vi "WS1050 Delta C Calculation.vi"(7 "WS1050/51":bool=TRUE, 8 "error in (no error)":errorcluster, 10 "DCap Target(pF)":dbl, 11 "Input":string[][](table)) -> (0 "error out":errorcluster, 1 "Total Bank Delta C(pF)":string[](array[string]), 2 "RTZ(pF)":string[][](array[string]), 3 "Delta C(pF)":string[][](array[string]), 4 "% Bank DeltaC":string[](array[string]))   [LabVIEW 2012]
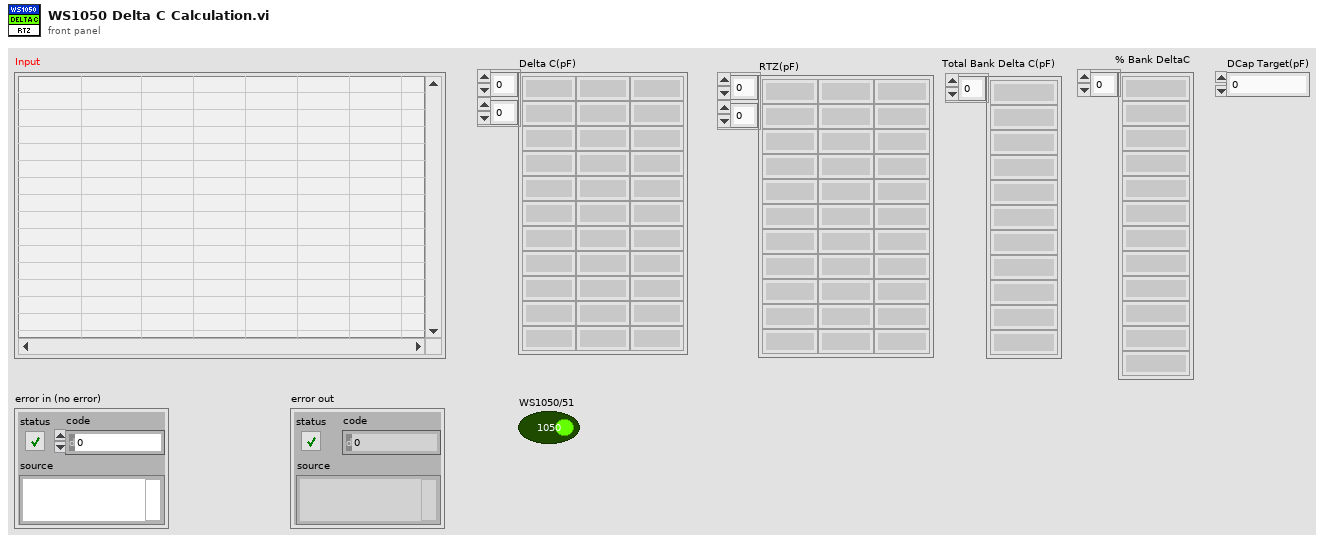
[diagram p1: front panel]
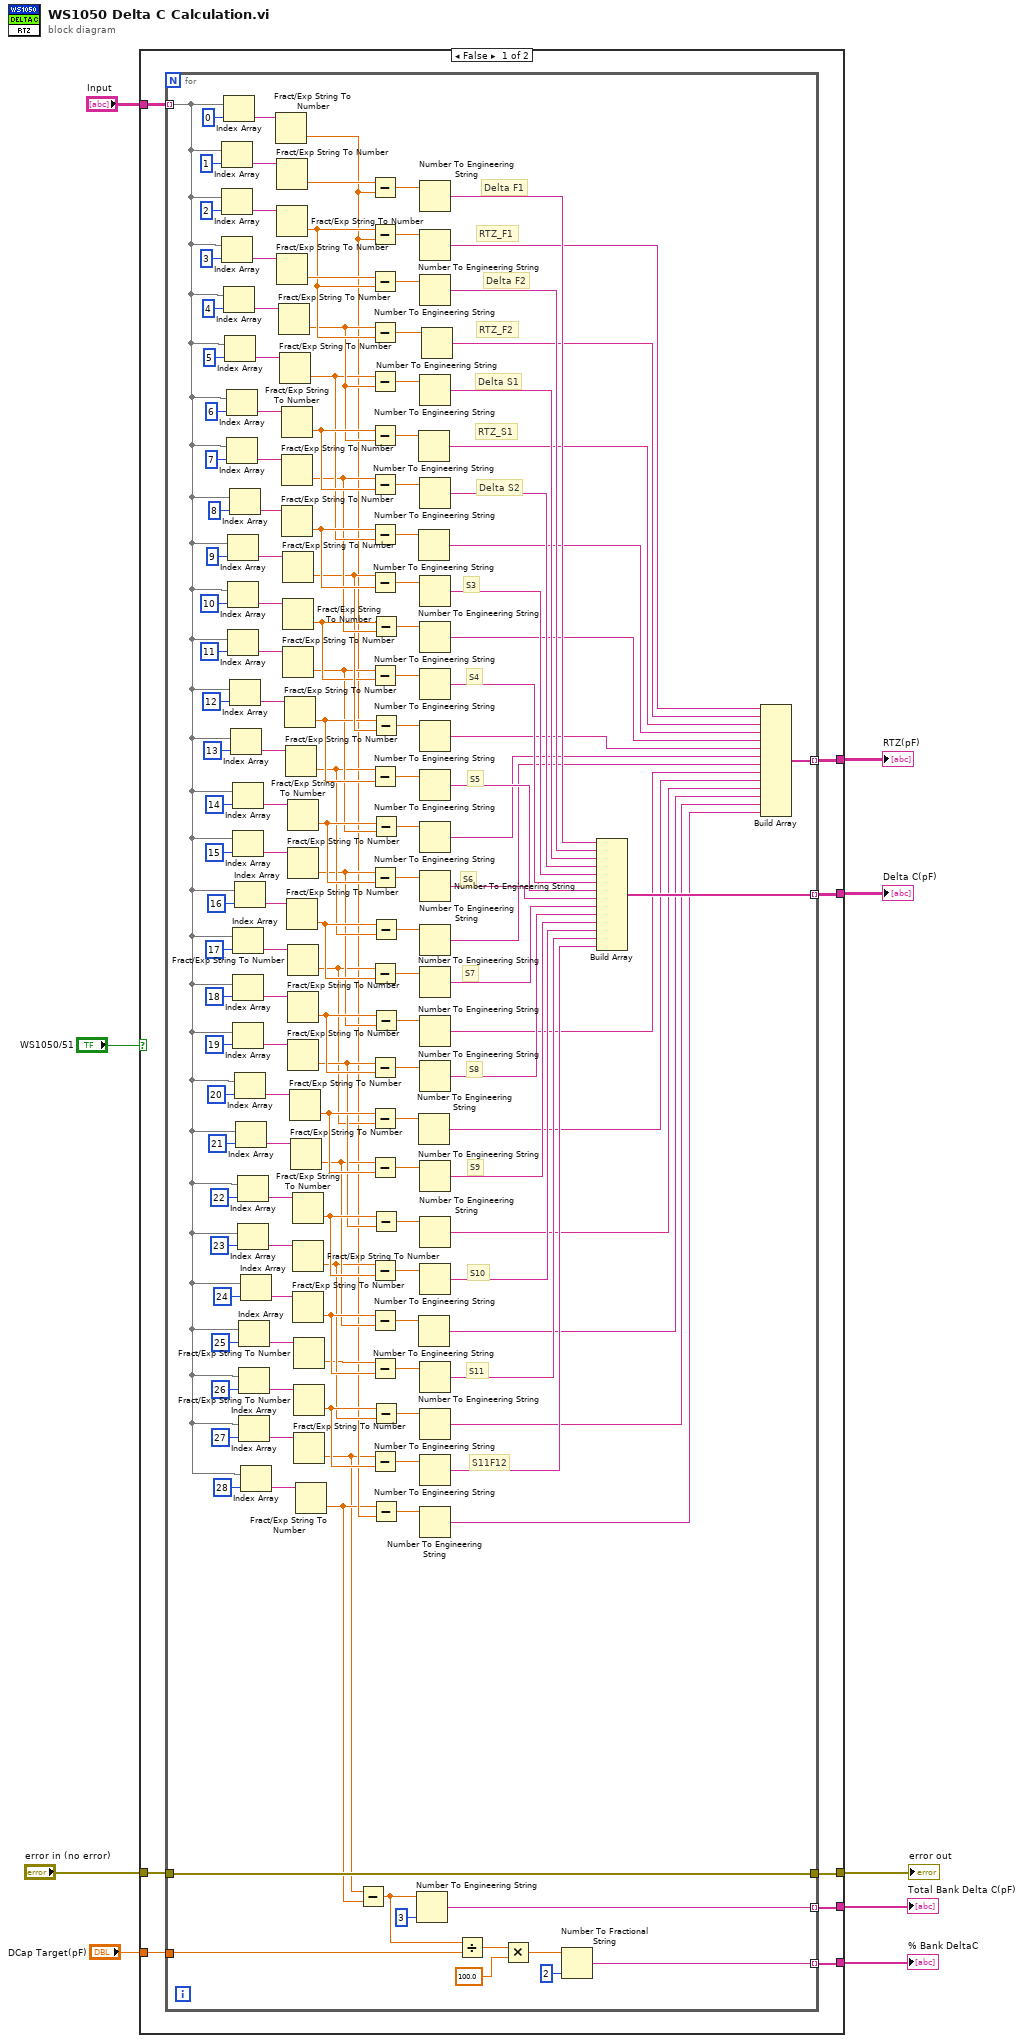
[diagram p0: block diagram]
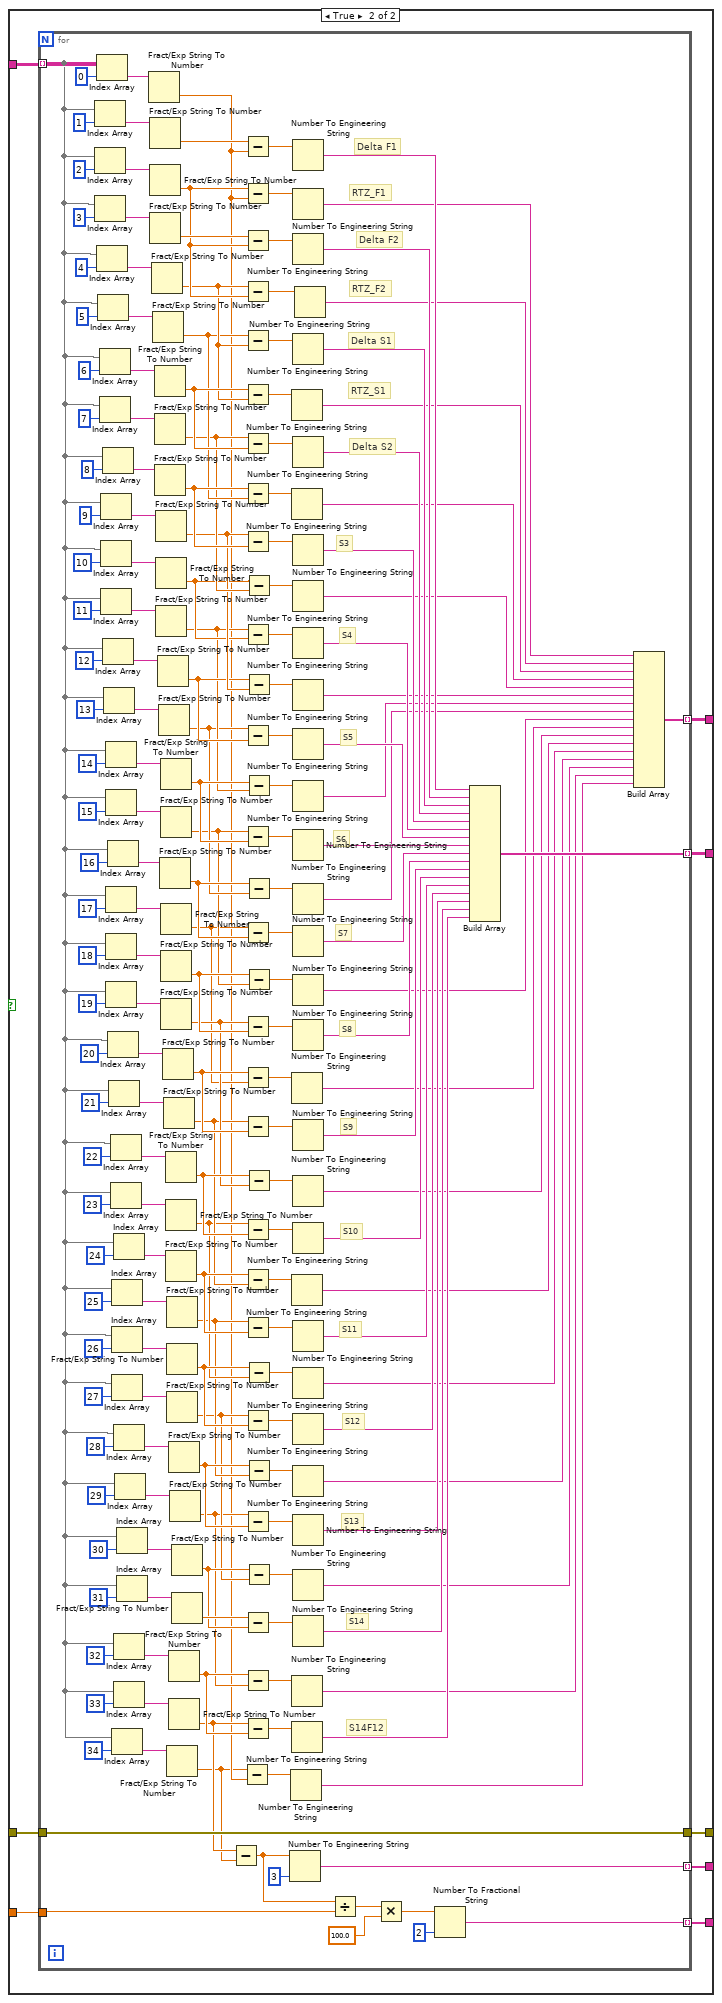
[diagram p2: hidden frame]
diagram:
  n1 = case shown="False" "WS1050/51" {
    tunnel: "Input" -> [w10 w181]
    tunnel: [w16 w180] -> w8
    tunnel: [w17 w179] -> w7
    tunnel: "error in (no error)" -> [w15 w178]
    tunnel: [w14 w177] -> w5
    tunnel: [w13 w176] -> w4
    tunnel: [w12 w175] -> w3
    tunnel: "DCap Target(pF)" -> [w11 w174]
    frame False {
      n2 = for {
        tunnel: w10 -> [w46] mode=indexing
        tunnel: [w85] -> w16 mode=indexing
        tunnel: [w31] -> w17 mode=indexing
        tunnel: w15 -> [w30]
        tunnel: [w30] -> w14
        tunnel: [w29] -> w13 mode=indexing
        tunnel: [w22] -> w12 mode=indexing
        tunnel: w11 -> [w21]
        # "RTZ_S1"
        # "RTZ_F2"
        # "RTZ_F1"
        # "S11F12"
        # "S11"
        # "S10"
        # "S9"
        # "S8"
        # "S7"
        # "S6"
        # "S5"
        # "S4"
        # "S3"
        # "Delta S2"
        # "Delta S1"
        # "Delta F2"
        # "Delta F1"
        n3 = Index Array(array=w46, index=1) -> (element=w168:string)
        n4 = Index Array(array=w46, index=2) -> (element=w167:string)
        n5 = Index Array(array=w46, index=3) -> (element=w164:string)
        n6 = Index Array(array=w46, index=0) -> (element=w169:string)
        n7 = Index Array(array=w46, index=4) -> (element=w163:string)
        n8 = Index Array(array=w46, index=5) -> (element=w160:string)
        n9 = Index Array(array=w46, index=6) -> (element=w159:string)
        n10 = Index Array(array=w46, index=7) -> (element=w156:string)
        n11 = Index Array(array=w46, index=9) -> (element=w143:string)
        n12 = Index Array(array=w46, index=10) -> (element=w144:string)
        n13 = Index Array(array=w46, index=11) -> (element=w147:string)
        n14 = Index Array(array=w46, index=8) -> (element=w142:string)
        n15 = Index Array(array=w46, index=12) -> (element=w148:string)
        n16 = Index Array(array=w46, index=13) -> (element=w151:string)
        n17 = Index Array(array=w46, index=14) -> (element=w152:string)
        n18 = Index Array(array=w46, index=15) -> (element=w155:string)
        n19 = Index Array(array=w46, index=17) -> (element=w96:string)
        n20 = Index Array(array=w46, index=18) -> (element=w97:string)
        n21 = Index Array(array=w46, index=19) -> (element=w100:string)
        n22 = Index Array(array=w46, index=16) -> (element=w95:string)
        n23 = Index Array(array=w46, index=20) -> (element=w101:string)
        n24 = Index Array(array=w46, index=21) -> (element=w104:string)
        n25 = Index Array(array=w46, index=22) -> (element=w105:string)
        n26 = Index Array(array=w46, index=23) -> (element=w108:string)
        n27 = Index Array(array=w46, index=25) -> (element=w115:string)
        n28 = Index Array(array=w46, index=26) -> (element=w114:string)
        n29 = Index Array(array=w46, index=27) -> (element=w111:string)
        n30 = Index Array(array=w46, index=24) -> (element=w116:string)
        n31 = Index Array(array=w46, index=28) -> (element=w110:string)
        n32 = Fract/Exp String To Number(string=w169) -> (number=w20:dbl)  [unwired: 3 in, 1 out]
        n33 = Fract/Exp String To Number(string=w168) -> (number=w171:dbl)  [unwired: 3 in, 1 out]
        n34 = Fract/Exp String To Number(string=w167) -> (number=w80:dbl)  [unwired: 3 in, 1 out]
        n35 = Fract/Exp String To Number(string=w164) -> (number=w138:dbl)  [unwired: 3 in, 1 out]
        n36 = Fract/Exp String To Number(string=w163) -> (number=w79:dbl)  [unwired: 3 in, 1 out]
        n37 = Fract/Exp String To Number(string=w160) -> (number=w76:dbl)  [unwired: 3 in, 1 out]
        n38 = Fract/Exp String To Number(string=w159) -> (number=w81:dbl)  [unwired: 3 in, 1 out]
        n39 = Fract/Exp String To Number(string=w156) -> (number=w74:dbl)  [unwired: 3 in, 1 out]
        n40 = Fract/Exp String To Number(string=w142) -> (number=w77:dbl)  [unwired: 3 in, 1 out]
        n41 = Fract/Exp String To Number(string=w143) -> (number=w72:dbl)  [unwired: 3 in, 1 out]
        n42 = Fract/Exp String To Number(string=w144) -> (number=w70:dbl)  [unwired: 3 in, 1 out]
        n43 = Fract/Exp String To Number(string=w147) -> (number=w58:dbl)  [unwired: 3 in, 1 out]
        n44 = Fract/Exp String To Number(string=w148) -> (number=w68:dbl)  [unwired: 3 in, 1 out]
        n45 = Fract/Exp String To Number(string=w151) -> (number=w57:dbl)  [unwired: 3 in, 1 out]
        n46 = Fract/Exp String To Number(string=w95) -> (number=w63:dbl)  [unwired: 3 in, 1 out]
        n47 = Fract/Exp String To Number(string=w152) -> (number=w66:dbl)  [unwired: 3 in, 1 out]
        n48 = Fract/Exp String To Number(string=w155) -> (number=w56:dbl)  [unwired: 3 in, 1 out]
        n49 = Fract/Exp String To Number(string=w96) -> (number=w55:dbl)  [unwired: 3 in, 1 out]
        n50 = Fract/Exp String To Number(string=w97) -> (number=w60:dbl)  [unwired: 3 in, 1 out]
        n51 = Fract/Exp String To Number(string=w100) -> (number=w59:dbl)  [unwired: 3 in, 1 out]
        n52 = Fract/Exp String To Number(string=w101) -> (number=w64:dbl)  [unwired: 3 in, 1 out]
        n53 = Fract/Exp String To Number(string=w104) -> (number=w52:dbl)  [unwired: 3 in, 1 out]
        n54 = Fract/Exp String To Number(string=w105) -> (number=w61:dbl)  [unwired: 3 in, 1 out]
        n55 = Fract/Exp String To Number(string=w108) -> (number=w49:dbl)  [unwired: 3 in, 1 out]
        n56 = Fract/Exp String To Number(string=w116) -> (number=w53:dbl)  [unwired: 3 in, 1 out]
        n57 = Fract/Exp String To Number(string=w115) -> (number=w47:dbl)  [unwired: 3 in, 1 out]
        n58 = Fract/Exp String To Number(string=w114) -> (number=w50:dbl)  [unwired: 3 in, 1 out]
        n59 = Fract/Exp String To Number(string=w111) -> (number=w18:dbl)  [unwired: 3 in, 1 out]
        n60 = Fract/Exp String To Number(string=w110) -> (number=w19:dbl)  [unwired: 3 in, 1 out]
        n61 = Subtract(x=w18, y=w19) -> (x-y=w27:dbl)
        n62 = Subtract(x=w171, y=w20) -> (x-y=w170:dbl)
        n63 = Subtract(x=w80, y=w20) -> (x-y=w84:dbl)
        n64 = Subtract(x=w138, y=w80) -> (x-y=w139:dbl)
        n65 = Subtract(x=w79, y=w80) -> (x-y=w83:dbl)
        n66 = Subtract(x=w76, y=w79) -> (x-y=w137:dbl)
        n67 = Subtract(x=w81, y=w79) -> (x-y=w82:dbl)
        n68 = Subtract(x=w74, y=w81) -> (x-y=w136:dbl)
        n69 = Subtract(x=w77, y=w76) -> (x-y=w78:dbl)
        n70 = Subtract(x=w72, y=w77) -> (x-y=w135:dbl)
        n71 = Subtract(x=w58, y=w70) -> (x-y=w134:dbl)
        n72 = Subtract(x=w57, y=w68) -> (x-y=w133:dbl)
        n73 = Subtract(x=w56, y=w66) -> (x-y=w132:dbl)
        n74 = Subtract(x=w55, y=w63) -> (x-y=w94:dbl)
        n75 = Subtract(x=w59, y=w60) -> (x-y=w119:dbl)
        n76 = Subtract(x=w64, y=w55) -> (x-y=w65:dbl)
        n77 = Subtract(x=w52, y=w64) -> (x-y=w120:dbl)
        n78 = Subtract(x=w49, y=w61) -> (x-y=w121:dbl)
        n79 = Subtract(x=w53, y=w52) -> (x-y=w54:dbl)
        n80 = Subtract(x=w47, y=w53) -> (x-y=w122:dbl)
        n81 = Subtract(x=w18, y=w50) -> (x-y=w123:dbl)
        n82 = Subtract(x=w70, y=w74) -> (x-y=w75:dbl)
        n83 = Subtract(x=w68, y=w72) -> (x-y=w73:dbl)
        n84 = Subtract(x=w66, y=w58) -> (x-y=w71:dbl)
        n85 = Subtract(x=w63, y=w57) -> (x-y=w69:dbl)
        n86 = Subtract(x=w60, y=w56) -> (x-y=w67:dbl)
        n87 = Subtract(x=w61, y=w59) -> (x-y=w62:dbl)
        n88 = Subtract(x=w50, y=w49) -> (x-y=w51:dbl)
        n89 = Subtract(x=w19, y=w20) -> (x-y=w48:dbl)
        n90 = Number To Engineering String(2:i16 3 ("precision (6)"), 4:w27) -> (0:w29:string)  [unwired: 2 in]
        n91 = Number To Engineering String(4:w82) -> (0:w43:string)  [unwired: 3 in]
        n92 = Number To Engineering String(4:w78) -> (0:w42:string)  [unwired: 3 in]
        n93 = Number To Engineering String(4:w65) -> (0:w36:string)  [unwired: 3 in]
        n94 = Number To Engineering String(4:w54) -> (0:w34:string)  [unwired: 3 in]
        n95 = Number To Engineering String(4:w170) -> (0:w131:string)  [unwired: 3 in]
        n96 = Number To Engineering String(4:w84) -> (0:w45:string)  [unwired: 3 in]
        n97 = Number To Engineering String(4:w139) -> (0:w130:string)  [unwired: 3 in]
        n98 = Number To Engineering String(4:w137) -> (0:w129:string)  [unwired: 3 in]
        n99 = Number To Engineering String(4:w136) -> (0:w128:string)  [unwired: 3 in]
        n100 = Number To Engineering String(4:w135) -> (0:w127:string)  [unwired: 3 in]
        n101 = Number To Engineering String(4:w75) -> (0:w41:string)  [unwired: 3 in]
        n102 = Number To Engineering String(4:w134) -> (0:w126:string)  [unwired: 3 in]
        n103 = Number To Engineering String(4:w73) -> (0:w40:string)  [unwired: 3 in]
        n104 = Number To Engineering String(4:w133) -> (0:w125:string)  [unwired: 3 in]
        n105 = Number To Engineering String(4:w71) -> (0:w39:string)  [unwired: 3 in]
        n106 = Number To Engineering String(4:w132) -> (0:w124:string)  [unwired: 3 in]
        n107 = Number To Engineering String(4:w69) -> (0:w38:string)  [unwired: 3 in]
        n108 = Number To Engineering String(4:w94) -> (0:w91:string)  [unwired: 3 in]
        n109 = Number To Engineering String(4:w67) -> (0:w37:string)  [unwired: 3 in]
        n110 = Number To Engineering String(4:w119) -> (0:w90:string)  [unwired: 3 in]
        n111 = Number To Engineering String(4:w120) -> (0:w89:string)  [unwired: 3 in]
        n112 = Number To Engineering String(4:w62) -> (0:w35:string)  [unwired: 3 in]
        n113 = Number To Engineering String(4:w121) -> (0:w88:string)  [unwired: 3 in]
        n114 = Number To Engineering String(4:w122) -> (0:w87:string)  [unwired: 3 in]
        n115 = Number To Engineering String(4:w51) -> (0:w33:string)  [unwired: 3 in]
        n116 = Number To Engineering String(4:w123) -> (0:w86:string)  [unwired: 3 in]
        n117 = Number To Engineering String(4:w48) -> (0:w32:string)  [unwired: 3 in]
        n118 = Number To Engineering String(4:w83) -> (0:w44:string)  [unwired: 3 in]
        n119 = Divide(x=w27, y=w21) -> (x/y=w26:dbl)
        n120 = Multiply(x=w26, y=100.0) -> (x*y=w24:dbl)
        n121 = Number To Fractional String(number=w24, precision (6)=i16 2) -> (F-format string=w22:string)  [unwired: 2 in]
        n122 = Build Array(w131, w130, w129, w128, w127, w126, w125, w124, w91, w90, w89, w88, w87, w86) -> (w85:string[])
        n123 = Build Array(w45, w44, w43, w42, w41, w40, w39, w38, w37, w36, w35, w34, w33, w32) -> (w31:string[])
      }
    }
    frame True {
      n124 = for {
        tunnel: w181 -> [w213] mode=indexing
        tunnel: [w262] -> w180 mode=indexing
        tunnel: [w195] -> w179 mode=indexing
        tunnel: w178 -> [w194]
        tunnel: [w194] -> w177
        tunnel: [w190] -> w176 mode=indexing
        tunnel: [w183] -> w175 mode=indexing
        tunnel: w174 -> [w182]
        # "RTZ_S1"
        # "RTZ_F2"
        # "RTZ_F1"
        # "S14F12"
        # "S14"
        # "S13"
        # "S12"
        # "S11"
        # "S10"
        # "S9"
        # "S8"
        # "S7"
        # "S6"
        # "S5"
        # "S4"
        # "S3"
        # "Delta S2"
        # "Delta S1"
        # "Delta F2"
        # "Delta F1"
        n125 = Index Array(array=w213, index=1) -> (element=w362:string)
        n126 = Index Array(array=w213, index=2) -> (element=w361:string)
        n127 = Index Array(array=w213, index=3) -> (element=w358:string)
        n128 = Index Array(array=w213, index=0) -> (element=w363:string)
        n129 = Index Array(array=w213, index=4) -> (element=w357:string)
        n130 = Index Array(array=w213, index=5) -> (element=w354:string)
        n131 = Index Array(array=w213, index=6) -> (element=w353:string)
        n132 = Index Array(array=w213, index=7) -> (element=w350:string)
        n133 = Index Array(array=w213, index=9) -> (element=w337:string)
        n134 = Index Array(array=w213, index=10) -> (element=w338:string)
        n135 = Index Array(array=w213, index=11) -> (element=w341:string)
        n136 = Index Array(array=w213, index=8) -> (element=w336:string)
        n137 = Index Array(array=w213, index=12) -> (element=w342:string)
        n138 = Index Array(array=w213, index=13) -> (element=w345:string)
        n139 = Index Array(array=w213, index=14) -> (element=w346:string)
        n140 = Index Array(array=w213, index=15) -> (element=w349:string)
        n141 = Index Array(array=w213, index=17) -> (element=w281:string)
        n142 = Index Array(array=w213, index=18) -> (element=w282:string)
        n143 = Index Array(array=w213, index=19) -> (element=w285:string)
        n144 = Index Array(array=w213, index=16) -> (element=w280:string)
        n145 = Index Array(array=w213, index=20) -> (element=w286:string)
        n146 = Index Array(array=w213, index=21) -> (element=w289:string)
        n147 = Index Array(array=w213, index=22) -> (element=w290:string)
        n148 = Index Array(array=w213, index=23) -> (element=w293:string)
        n149 = Index Array(array=w213, index=25) -> (element=w306:string)
        n150 = Index Array(array=w213, index=26) -> (element=w305:string)
        n151 = Index Array(array=w213, index=27) -> (element=w302:string)
        n152 = Index Array(array=w213, index=34) -> (element=w214:string)
        n153 = Index Array(array=w213, index=24) -> (element=w307:string)
        n154 = Index Array(array=w213, index=28) -> (element=w301:string)
        n155 = Index Array(array=w213, index=32) -> (element=w273:string)
        n156 = Index Array(array=w213, index=33) -> (element=w276:string)
        n157 = Index Array(array=w213, index=29) -> (element=w298:string)
        n158 = Index Array(array=w213, index=30) -> (element=w297:string)
        n159 = Index Array(array=w213, index=31) -> (element=w294:string)
        n160 = Fract/Exp String To Number(string=w363) -> (number=w192:dbl)  [unwired: 3 in, 1 out]
        n161 = Fract/Exp String To Number(string=w362) -> (number=w365:dbl)  [unwired: 3 in, 1 out]
        n162 = Fract/Exp String To Number(string=w361) -> (number=w257:dbl)  [unwired: 3 in, 1 out]
        n163 = Fract/Exp String To Number(string=w358) -> (number=w332:dbl)  [unwired: 3 in, 1 out]
        n164 = Fract/Exp String To Number(string=w357) -> (number=w256:dbl)  [unwired: 3 in, 1 out]
        n165 = Fract/Exp String To Number(string=w354) -> (number=w253:dbl)  [unwired: 3 in, 1 out]
        n166 = Fract/Exp String To Number(string=w353) -> (number=w258:dbl)  [unwired: 3 in, 1 out]
        n167 = Fract/Exp String To Number(string=w350) -> (number=w251:dbl)  [unwired: 3 in, 1 out]
        n168 = Fract/Exp String To Number(string=w336) -> (number=w254:dbl)  [unwired: 3 in, 1 out]
        n169 = Fract/Exp String To Number(string=w337) -> (number=w249:dbl)  [unwired: 3 in, 1 out]
        n170 = Fract/Exp String To Number(string=w338) -> (number=w247:dbl)  [unwired: 3 in, 1 out]
        n171 = Fract/Exp String To Number(string=w341) -> (number=w235:dbl)  [unwired: 3 in, 1 out]
        n172 = Fract/Exp String To Number(string=w342) -> (number=w245:dbl)  [unwired: 3 in, 1 out]
        n173 = Fract/Exp String To Number(string=w345) -> (number=w234:dbl)  [unwired: 3 in, 1 out]
        n174 = Fract/Exp String To Number(string=w280) -> (number=w240:dbl)  [unwired: 3 in, 1 out]
        n175 = Fract/Exp String To Number(string=w346) -> (number=w243:dbl)  [unwired: 3 in, 1 out]
        n176 = Fract/Exp String To Number(string=w349) -> (number=w233:dbl)  [unwired: 3 in, 1 out]
        n177 = Fract/Exp String To Number(string=w281) -> (number=w232:dbl)  [unwired: 3 in, 1 out]
        n178 = Fract/Exp String To Number(string=w282) -> (number=w237:dbl)  [unwired: 3 in, 1 out]
        n179 = Fract/Exp String To Number(string=w285) -> (number=w236:dbl)  [unwired: 3 in, 1 out]
        n180 = Fract/Exp String To Number(string=w286) -> (number=w241:dbl)  [unwired: 3 in, 1 out]
        n181 = Fract/Exp String To Number(string=w289) -> (number=w229:dbl)  [unwired: 3 in, 1 out]
        n182 = Fract/Exp String To Number(string=w290) -> (number=w238:dbl)  [unwired: 3 in, 1 out]
        n183 = Fract/Exp String To Number(string=w293) -> (number=w226:dbl)  [unwired: 3 in, 1 out]
        n184 = Fract/Exp String To Number(string=w307) -> (number=w230:dbl)  [unwired: 3 in, 1 out]
        n185 = Fract/Exp String To Number(string=w306) -> (number=w223:dbl)  [unwired: 3 in, 1 out]
        n186 = Fract/Exp String To Number(string=w305) -> (number=w227:dbl)  [unwired: 3 in, 1 out]
        n187 = Fract/Exp String To Number(string=w302) -> (number=w220:dbl)  [unwired: 3 in, 1 out]
        n188 = Fract/Exp String To Number(string=w214) -> (number=w191:dbl)  [unwired: 3 in, 1 out]
        n189 = Fract/Exp String To Number(string=w301) -> (number=w224:dbl)  [unwired: 3 in, 1 out]
        n190 = Fract/Exp String To Number(string=w273) -> (number=w218:dbl)  [unwired: 3 in, 1 out]
        n191 = Fract/Exp String To Number(string=w276) -> (number=w193:dbl)  [unwired: 3 in, 1 out]
        n192 = Fract/Exp String To Number(string=w298) -> (number=w217:dbl)  [unwired: 3 in, 1 out]
        n193 = Fract/Exp String To Number(string=w297) -> (number=w221:dbl)  [unwired: 3 in, 1 out]
        n194 = Fract/Exp String To Number(string=w294) -> (number=w317:dbl)  [unwired: 3 in, 1 out]
        n195 = Subtract(x=w193, y=w191) -> (x-y=w188:dbl)
        n196 = Subtract(x=w191, y=w192) -> (x-y=w216:dbl)
        n197 = Subtract(x=w365, y=w192) -> (x-y=w364:dbl)
        n198 = Subtract(x=w257, y=w192) -> (x-y=w261:dbl)
        n199 = Subtract(x=w332, y=w257) -> (x-y=w333:dbl)
        n200 = Subtract(x=w256, y=w257) -> (x-y=w260:dbl)
        n201 = Subtract(x=w253, y=w256) -> (x-y=w331:dbl)
        n202 = Subtract(x=w258, y=w256) -> (x-y=w259:dbl)
        n203 = Subtract(x=w251, y=w258) -> (x-y=w330:dbl)
        n204 = Subtract(x=w254, y=w253) -> (x-y=w255:dbl)
        n205 = Subtract(x=w249, y=w254) -> (x-y=w329:dbl)
        n206 = Subtract(x=w235, y=w247) -> (x-y=w328:dbl)
        n207 = Subtract(x=w234, y=w245) -> (x-y=w327:dbl)
        n208 = Subtract(x=w233, y=w243) -> (x-y=w326:dbl)
        n209 = Subtract(x=w232, y=w240) -> (x-y=w279:dbl)
        n210 = Subtract(x=w236, y=w237) -> (x-y=w310:dbl)
        n211 = Subtract(x=w241, y=w232) -> (x-y=w242:dbl)
        n212 = Subtract(x=w229, y=w241) -> (x-y=w311:dbl)
        n213 = Subtract(x=w226, y=w238) -> (x-y=w312:dbl)
        n214 = Subtract(x=w230, y=w229) -> (x-y=w231:dbl)
        n215 = Subtract(x=w223, y=w230) -> (x-y=w313:dbl)
        n216 = Subtract(x=w220, y=w227) -> (x-y=w314:dbl)
        n217 = Subtract(x=w217, y=w224) -> (x-y=w315:dbl)
        n218 = Subtract(x=w317, y=w221) -> (x-y=w316:dbl)
        n219 = Subtract(x=w218, y=w217) -> (x-y=w219:dbl)
        n220 = Subtract(x=w193, y=w218) -> (x-y=w272:dbl)
        n221 = Subtract(x=w247, y=w251) -> (x-y=w252:dbl)
        n222 = Subtract(x=w245, y=w249) -> (x-y=w250:dbl)
        n223 = Subtract(x=w243, y=w235) -> (x-y=w248:dbl)
        n224 = Subtract(x=w240, y=w234) -> (x-y=w246:dbl)
        n225 = Subtract(x=w237, y=w233) -> (x-y=w244:dbl)
        n226 = Subtract(x=w238, y=w236) -> (x-y=w239:dbl)
        n227 = Subtract(x=w227, y=w226) -> (x-y=w228:dbl)
        n228 = Subtract(x=w224, y=w223) -> (x-y=w225:dbl)
        n229 = Subtract(x=w221, y=w220) -> (x-y=w222:dbl)
        n230 = Number To Engineering String(2:i16 3 ("precision (6)"), 4:w188) -> (0:w190:string)  [unwired: 2 in]
        n231 = Number To Engineering String(4:w216) -> (0:w196:string)  [unwired: 3 in]
        n232 = Number To Engineering String(4:w259) -> (0:w210:string)  [unwired: 3 in]
        n233 = Number To Engineering String(4:w255) -> (0:w209:string)  [unwired: 3 in]
        n234 = Number To Engineering String(4:w242) -> (0:w203:string)  [unwired: 3 in]
        n235 = Number To Engineering String(4:w231) -> (0:w201:string)  [unwired: 3 in]
        n236 = Number To Engineering String(4:w219) -> (0:w197:string)  [unwired: 3 in]
        n237 = Number To Engineering String(4:w272) -> (0:w263:string)  [unwired: 3 in]
        n238 = Number To Engineering String(4:w364) -> (0:w325:string)  [unwired: 3 in]
        n239 = Number To Engineering String(4:w261) -> (0:w212:string)  [unwired: 3 in]
        n240 = Number To Engineering String(4:w333) -> (0:w324:string)  [unwired: 3 in]
        n241 = Number To Engineering String(4:w331) -> (0:w323:string)  [unwired: 3 in]
        n242 = Number To Engineering String(4:w330) -> (0:w322:string)  [unwired: 3 in]
        n243 = Number To Engineering String(4:w329) -> (0:w321:string)  [unwired: 3 in]
        n244 = Number To Engineering String(4:w252) -> (0:w208:string)  [unwired: 3 in]
        n245 = Number To Engineering String(4:w328) -> (0:w320:string)  [unwired: 3 in]
        n246 = Number To Engineering String(4:w250) -> (0:w207:string)  [unwired: 3 in]
        n247 = Number To Engineering String(4:w327) -> (0:w319:string)  [unwired: 3 in]
        n248 = Number To Engineering String(4:w248) -> (0:w206:string)  [unwired: 3 in]
        n249 = Number To Engineering String(4:w326) -> (0:w318:string)  [unwired: 3 in]
        n250 = Number To Engineering String(4:w246) -> (0:w205:string)  [unwired: 3 in]
        n251 = Number To Engineering String(4:w279) -> (0:w271:string)  [unwired: 3 in]
        n252 = Number To Engineering String(4:w244) -> (0:w204:string)  [unwired: 3 in]
        n253 = Number To Engineering String(4:w310) -> (0:w270:string)  [unwired: 3 in]
        n254 = Number To Engineering String(4:w311) -> (0:w269:string)  [unwired: 3 in]
        n255 = Number To Engineering String(4:w239) -> (0:w202:string)  [unwired: 3 in]
        n256 = Number To Engineering String(4:w312) -> (0:w268:string)  [unwired: 3 in]
        n257 = Number To Engineering String(4:w313) -> (0:w267:string)  [unwired: 3 in]
        n258 = Number To Engineering String(4:w228) -> (0:w200:string)  [unwired: 3 in]
        n259 = Number To Engineering String(4:w314) -> (0:w266:string)  [unwired: 3 in]
        n260 = Number To Engineering String(4:w225) -> (0:w199:string)  [unwired: 3 in]
        n261 = Number To Engineering String(4:w315) -> (0:w265:string)  [unwired: 3 in]
        n262 = Number To Engineering String(4:w222) -> (0:w198:string)  [unwired: 3 in]
        n263 = Number To Engineering String(4:w316) -> (0:w264:string)  [unwired: 3 in]
        n264 = Number To Engineering String(4:w260) -> (0:w211:string)  [unwired: 3 in]
        n265 = Divide(x=w188, y=w182) -> (x/y=w187:dbl)
        n266 = Multiply(x=w187, y=100.0) -> (x*y=w185:dbl)
        n267 = Number To Fractional String(number=w185, precision (6)=i16 2) -> (F-format string=w183:string)  [unwired: 2 in]
        n268 = Build Array(w325, w324, w323, w322, w321, w320, w319, w318, w271, w270, w269, w268, w267, w266, w265, w264, w263) -> (w262:string[])
        n269 = Build Array(w212, w211, w210, w209, w208, w207, w206, w205, w204, w203, w202, w201, w200, w199, w198, w197, w196) -> (w195:string[])
      }
    }
  }
  "Delta C(pF)" <- w8
  "RTZ(pF)" <- w7
  "error out" <- w5
  "Total Bank Delta C(pF)" <- w4
  "% Bank DeltaC" <- w3
